vi "Write VS Values to Driver.vi"(8 "error in":errorcluster, 10 "VS Values":dbl[](array[numeric]), 11 "Signal Indices In":i32[](array[numeric])) -> (0 "error out":errorcluster)   [LabVIEW 2026, in "Runtime Configuration Support Inline Async Example Custom Device Engine.lvlib"]
uses:
  Runtime Configuration Support Inline Async Example Custom Device Engine.lvlib
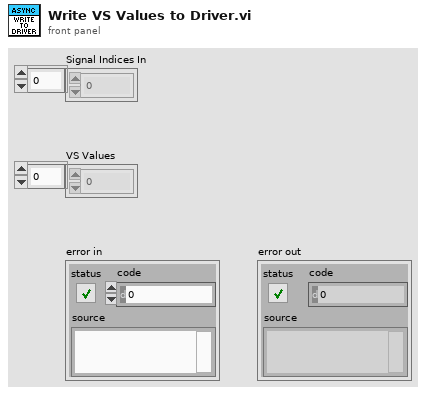
[diagram p1: front panel]
types:
  T1 = enum16{"Initialize", "Set In Val", "Get In Val", "Set Block", "Set Out Val", "Get Out Val", "Get In Array", "Get Out Array"}
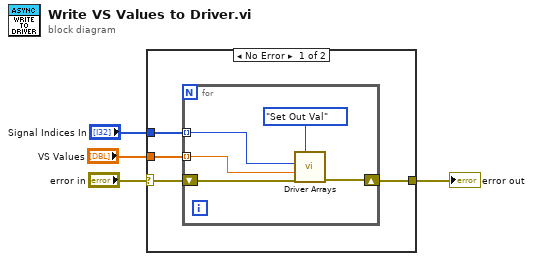
[diagram p0: block diagram]
diagram:
  n1 = case shown="No Error" "error in" {
    selector: "error in" -> [w7 w14]
    tunnel: "Signal Indices In" -> [w6 _]
    tunnel: "VS Values" -> [w5 _]
    tunnel: [w8 w14] -> w4
    frame No Error {
      n2 = for {
        shift-right: [w12] -> w8
        shift-left: w7 -> [w13]
        tunnel: w6 -> [w10] mode=indexing
        tunnel: w5 -> [w9] mode=indexing
        n3 = call "Driver Arrays.vi"("error in"=w13, "Value"=w9, "Index"=w10, "Curr Operation"=T1."Set Out Val") -> ("error out"=w12:errorcluster)  [unwired: 4 in, 3 out]
      }
    }
    frame Error {
    }
  }
  "error out" <- w4
